vi "control gas flow.vi"(5 "gas flow, %":dbl=11.0, 6 "action":T2(ring)=enum."stop UP/DOWN", 7 "heater":dbl=11.0, 8 "gas flow":refnum<vi>, 10 "seconds":i32=1) -> (0 "gas flow out":T1={"ramp DOWN time step (sec)"=120, "DOWN step (%)"=3.0, "last check (min)"=3, "heater below"=TRUE, "heater above"=FALSE, "check every # min"=11.0, "upper"=12.0, "lower"=3.0, "heater"=0.0, "heater in range"=FALSE, "(total # of ramp DOWN steps)"=30, "ramp step (%)"=0.1, "DOWN time (min)"=60.0, "UP time (min)"=60.0, "(total # of ramp UP steps)"=30, "UP step (%)"=3.0, "ramp UP time step (sec)"=120, "set gas"=FALSE, "to"=90.0, "ramp UP"=FALSE, "ramp DOWN"=FALSE, "ramp UP steps so far"=2, "ramp UP in progress"=FALSE, "ramp DOWN steps so far "=0, "ramp DOWN in progress"=FALSE, "idle"=FALSE, "Gas flow, %"=90.0, "Control Gas"=FALSE, "state"=enum."ramp down"} {"Gas flow, %" format="%.2f"; "heater" format="%.2f"})   [LabVIEW 2010]
uses:
  gas flow control.ctl
  itc 503 box - control.ctl
panel:
  in  "gas flow control":T1={"ramp DOWN time step (sec)"=120, "DOWN step (%)"=3.0, "last check (min)"=3, "heater below"=TRUE, "heater above"=FALSE, "check every # min"=11.0, "upper"=12.0, "lower"=3.0, "heater"=0.0, "heater in range"=FALSE, "(total # of ramp DOWN steps)"=30, "ramp step (%)"=0.1, "DOWN time (min)"=60.0, "UP time (min)"=60.0, "(total # of ramp UP steps)"=30, "UP step (%)"=3.0, "ramp UP time step (sec)"=120, "set gas"=FALSE, "to"=90.0, "ramp UP"=FALSE, "ramp DOWN"=FALSE, "ramp UP steps so far"=2, "ramp UP in progress"=FALSE, "ramp DOWN steps so far "=0, "ramp DOWN in progress"=FALSE, "idle"=FALSE, "Gas flow, %"=90.0, "Control Gas"=FALSE, "state"=enum."ramp down"} {"Gas flow, %" format="%.2f"; "heater" format="%.2f"}
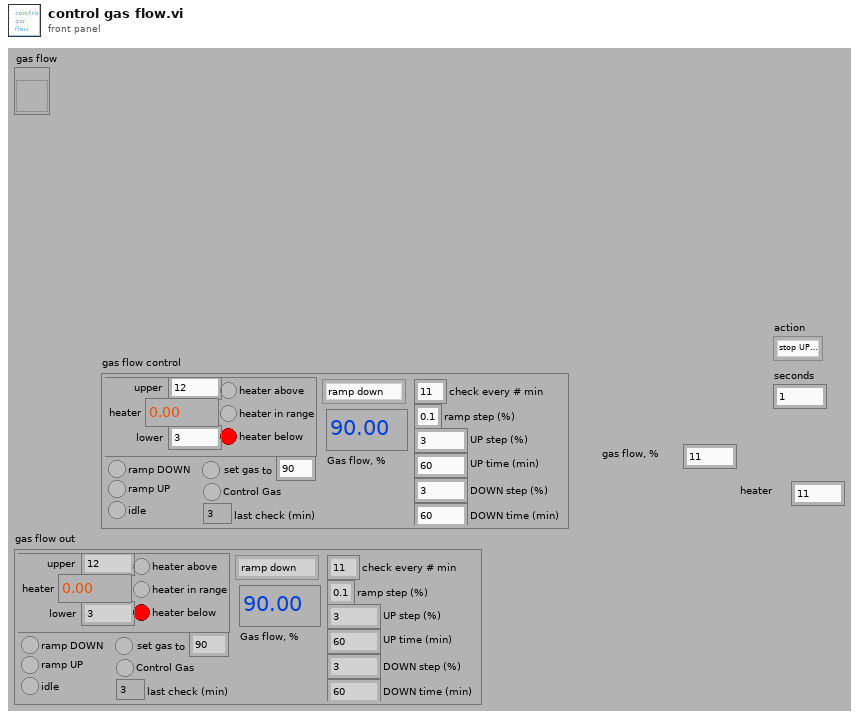
[diagram p1: front panel]
types:
  T1 = typedef "gas flow control.ctl" = cluster{"ramp DOWN time step (sec)":i32, "DOWN step (%)":dbl, "last check (min)":i32, "heater below":bool, "heater above":bool, "check every # min":dbl, "upper":dbl, "lower":dbl, "heater":dbl, "heater in range":bool, "(total # of ramp DOWN steps)":i32, "ramp step (%)":dbl, "DOWN time (min)":dbl, "UP time (min)":dbl, "(total # of ramp UP steps)":i32, "UP step (%)":dbl, "ramp UP time step (sec)":i32, "set gas":bool, "to":dbl, "ramp UP":bool, "ramp DOWN":bool, "ramp UP steps so far":i32, "ramp UP in progress":bool, "ramp DOWN steps so far ":i32, "ramp DOWN in progress":bool, "idle":bool, "Gas flow, %":dbl, "Control Gas":bool, "state":enum16{"normal", "ramp up", "ramp down"}}
  T2 = enum16{"check", "force UP", "stop UP/DOWN", "force DOWN", "init", "set gas to", "turn off", "turn on", "update parameters"}
  T3 = typedef "itc 503 box - control.ctl" = enum16{"heater manual and zero", "heater auto", "upload D", "upload I", "upload P", "shut off", "init", "read sweep table", "disable", "enable", "read state", "set gas to", "stop sweep", "start sweep", "test", "set temperature to", "write sweep table"}
  T4 = cluster{"ramp DOWN time step (sec)":i32, "DOWN step (%)":dbl, "last check (min)":i32, "heater below":bool, "heater above":bool, "check every # min":dbl, "upper":dbl, "lower":dbl, "heater":dbl, "heater in range":bool, "(total # of ramp DOWN steps)":i32, "ramp step (%)":dbl, "DOWN time (min)":dbl, "UP time (min)":dbl, "(total # of ramp UP steps)":i32, "UP step (%)":dbl, "ramp UP time step (sec)":i32, "set gas":bool, "to":dbl, "ramp UP":bool, "ramp DOWN":bool, "ramp UP steps so far":i32, "ramp UP in progress":bool, "ramp DOWN steps so far ":i32, "ramp DOWN in progress":bool, "idle":bool, "Gas flow, %":dbl, "Control Gas":bool, "state":enum16{"normal", "ramp up", "ramp down"}}
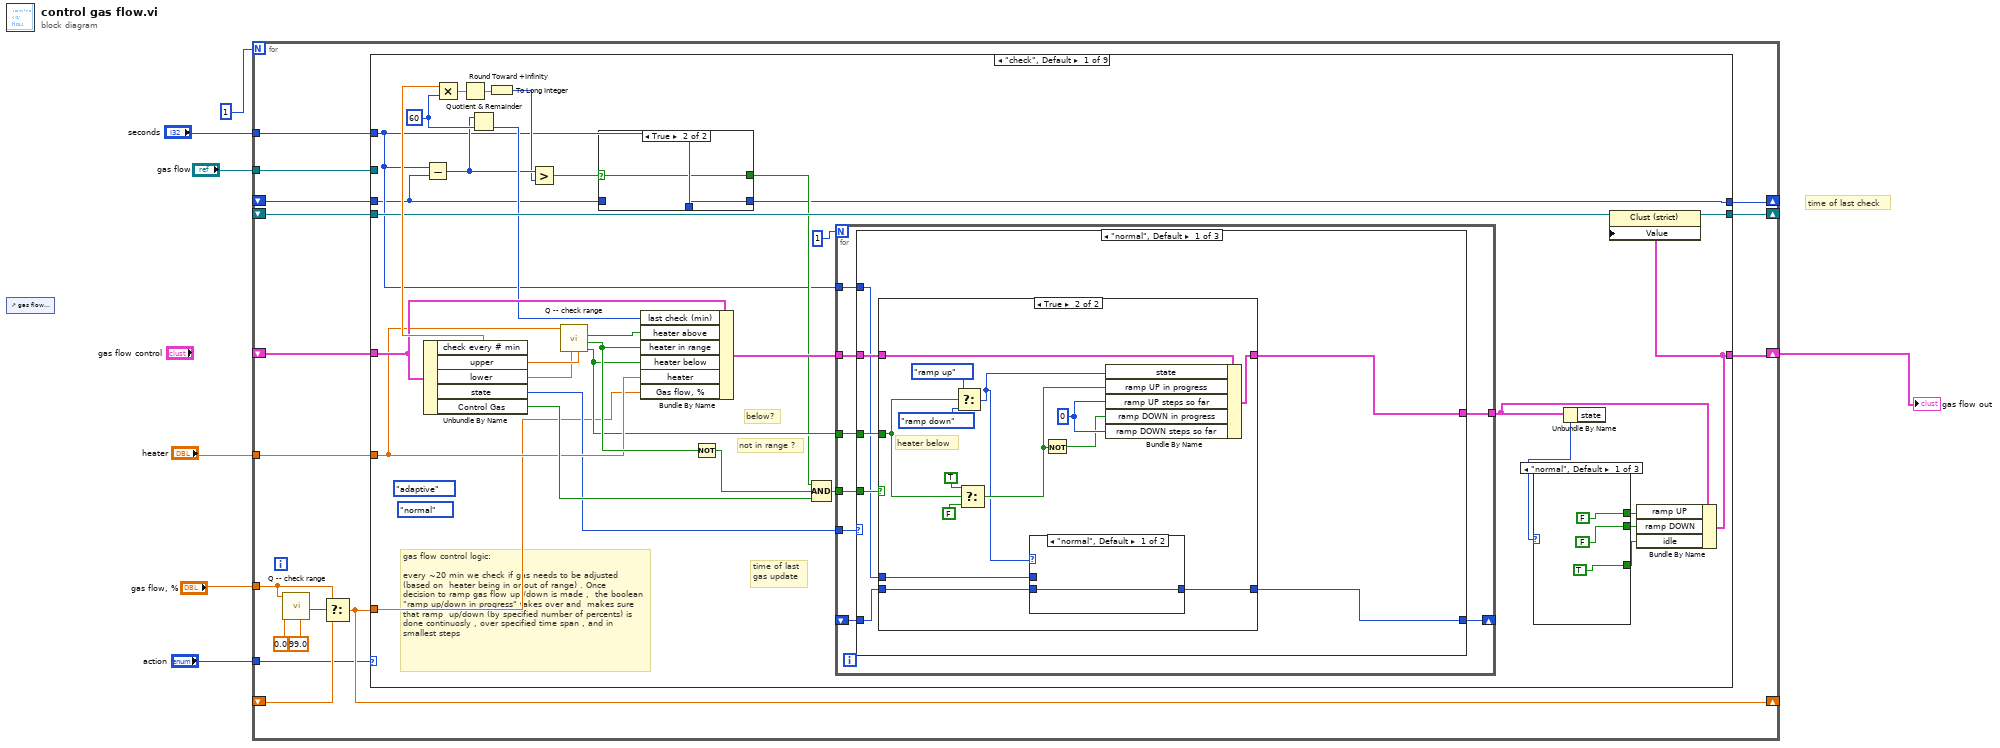
[diagram p0: block diagram]
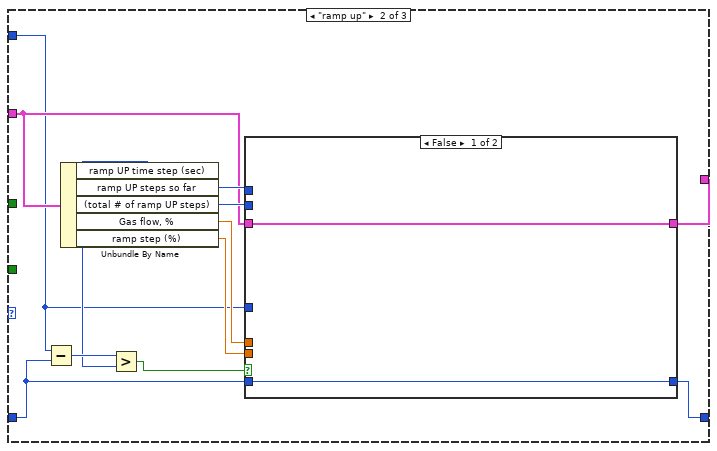
[diagram p4: hidden frame]
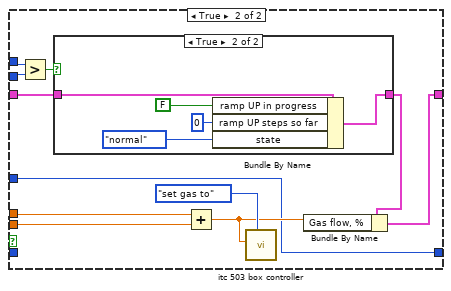
[diagram p5: hidden frame]
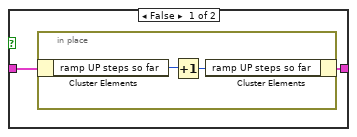
[diagram p6: hidden frame]
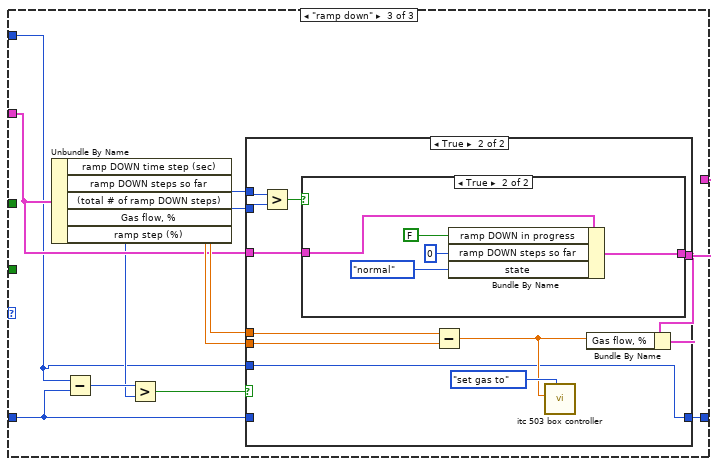
[diagram p7: hidden frame]
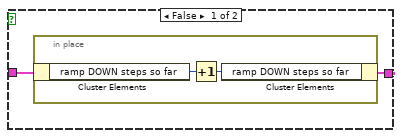
[diagram p9: hidden frame]
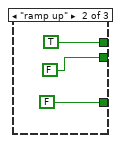
[diagram p11: hidden frame]
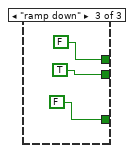
[diagram p12: hidden frame]
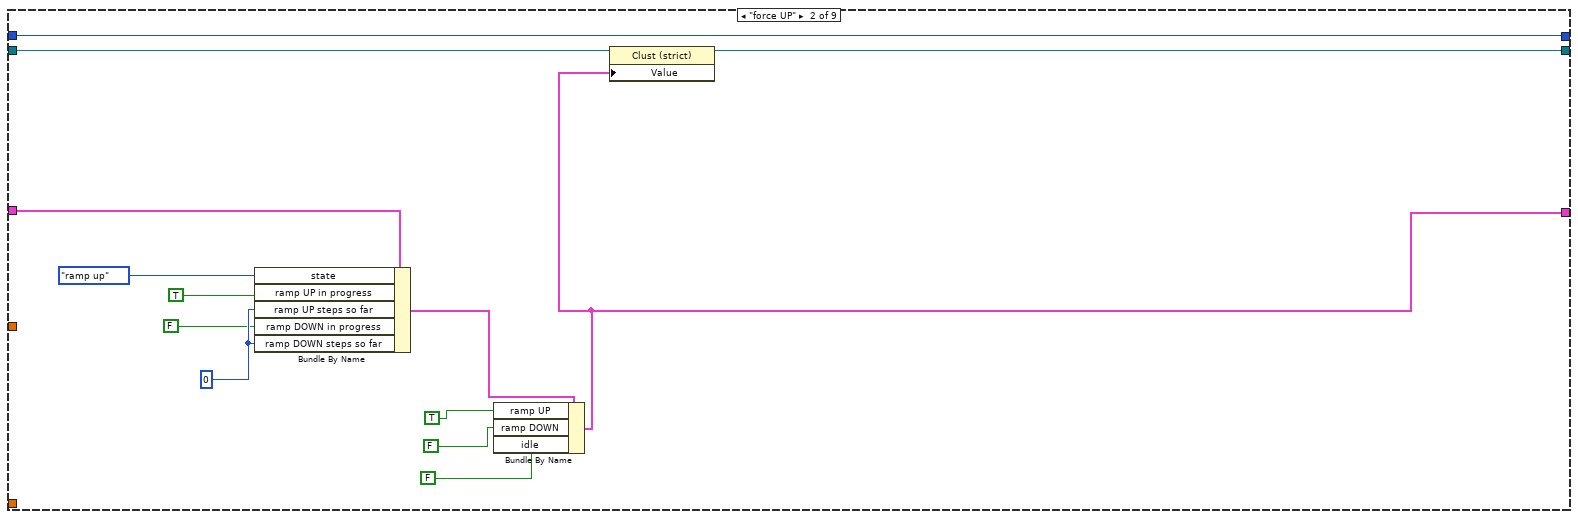
[diagram p13: hidden frame]
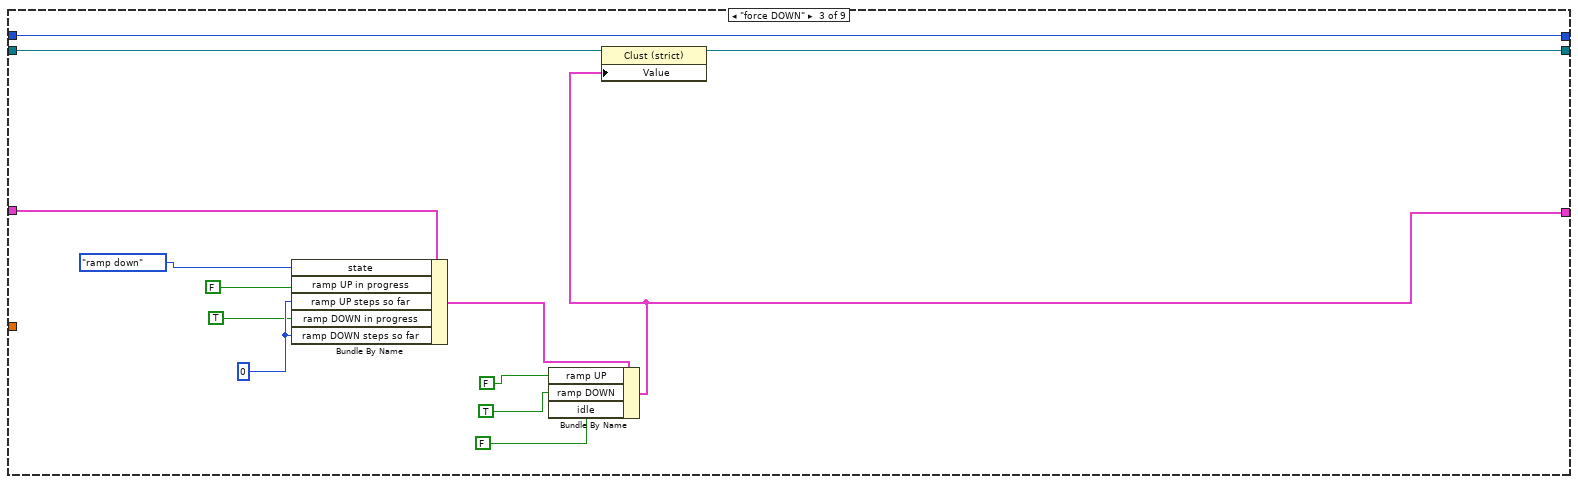
[diagram p14: hidden frame]
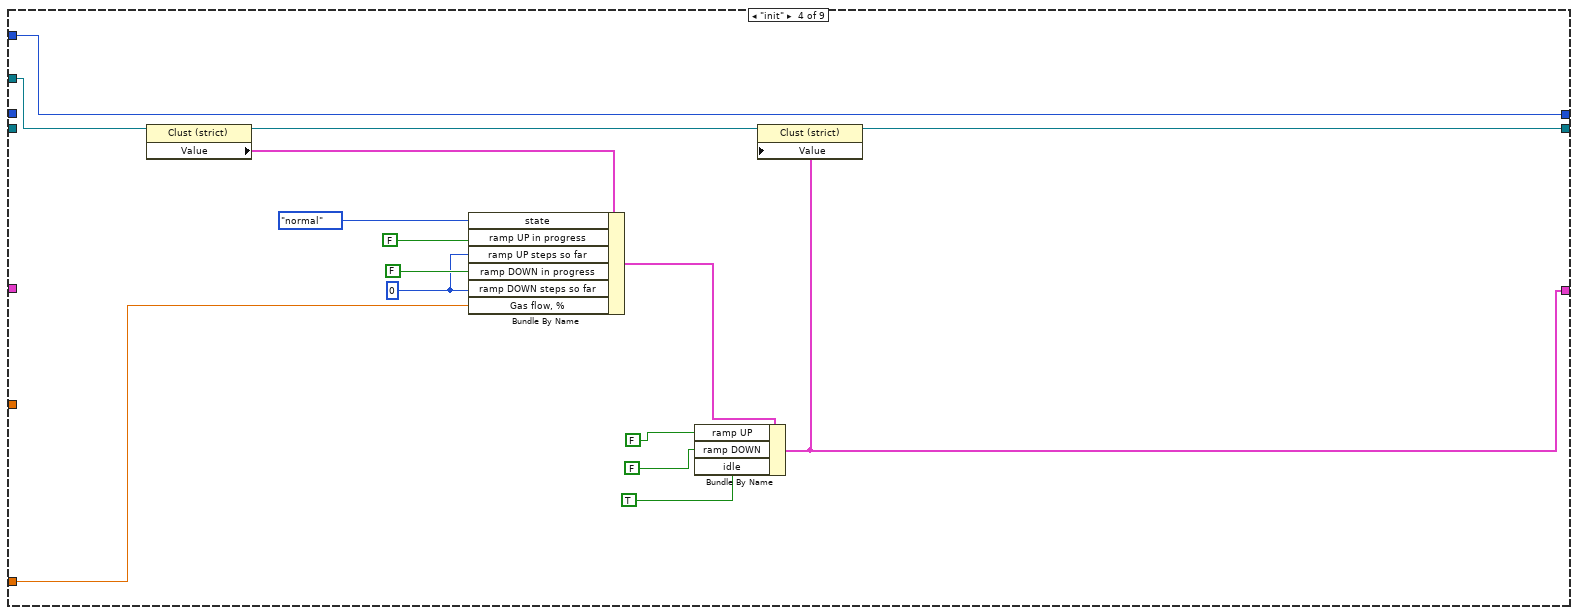
[diagram p15: hidden frame]
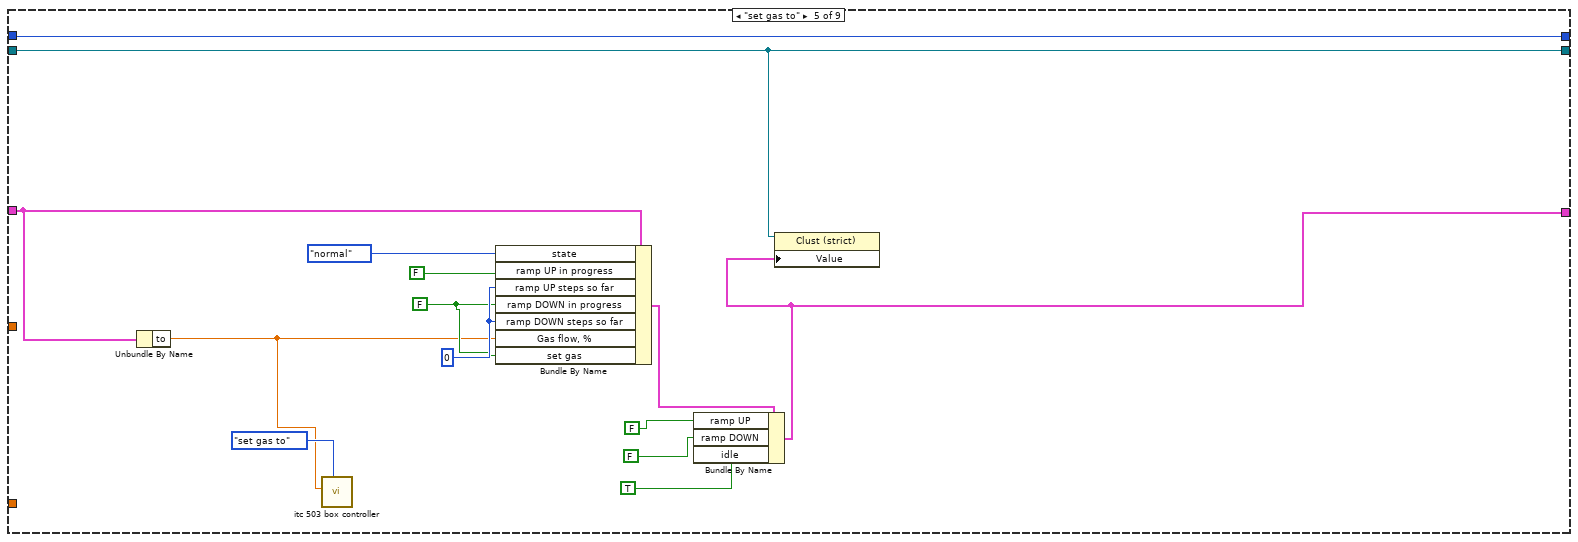
[diagram p16: hidden frame]
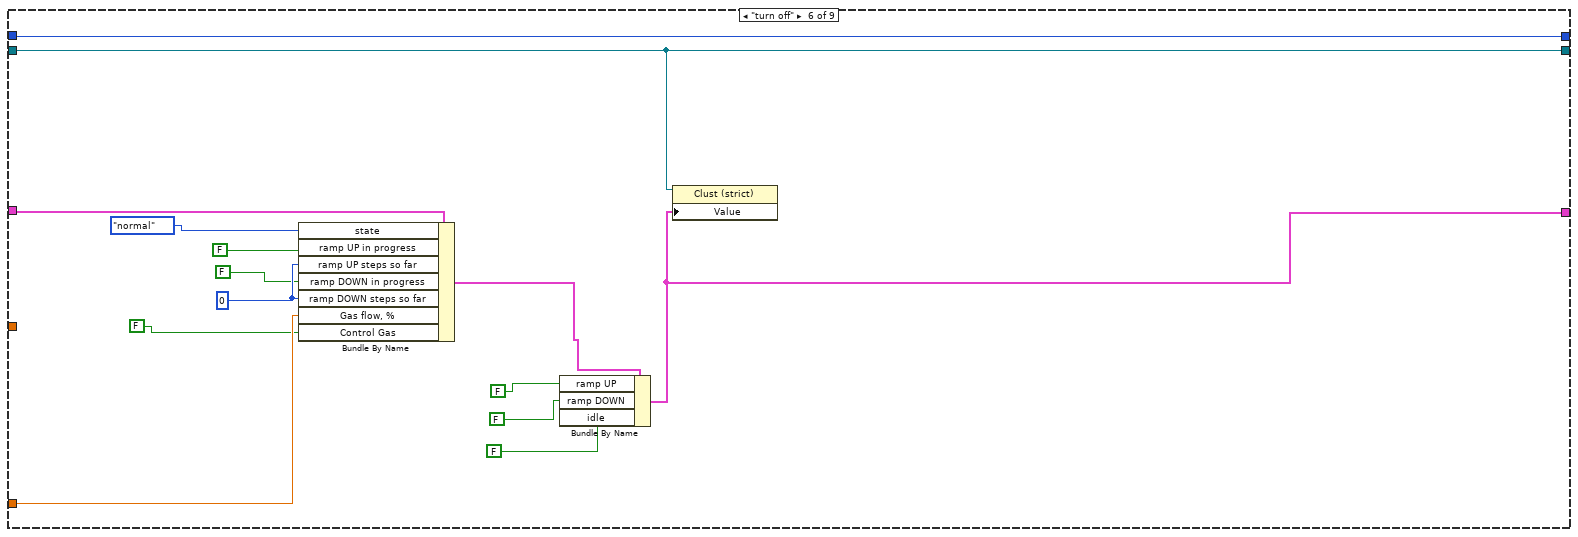
[diagram p17: hidden frame]
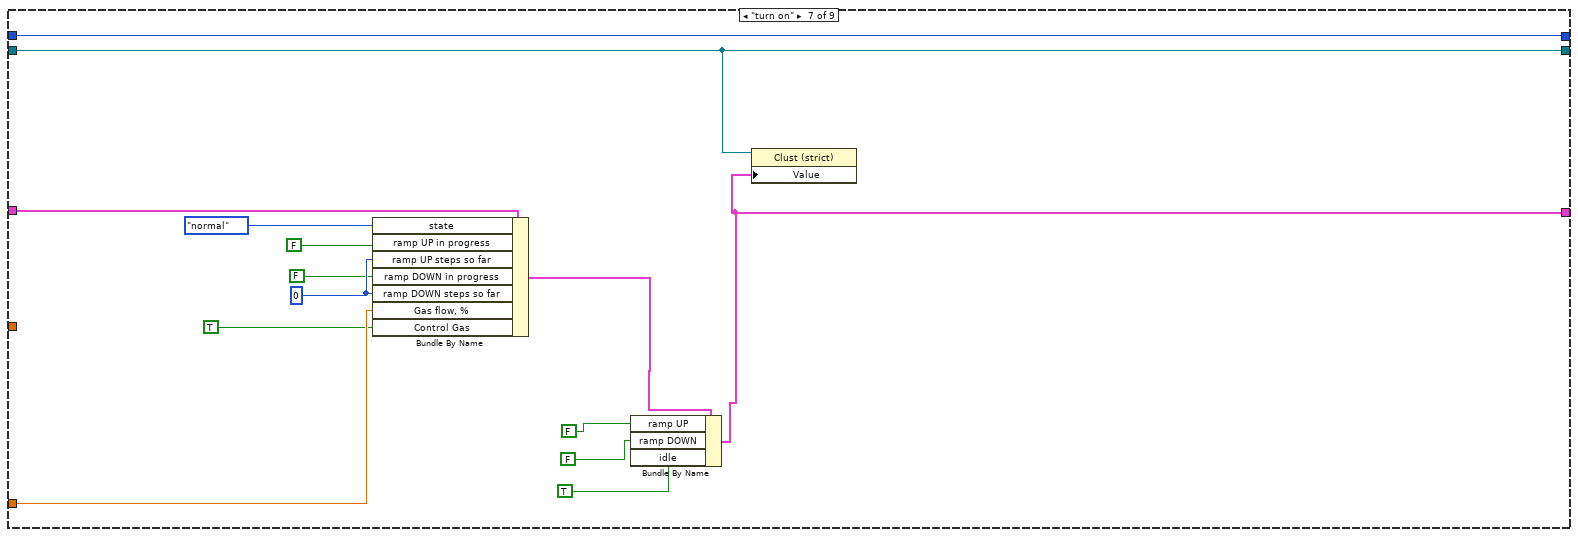
[diagram p18: hidden frame]
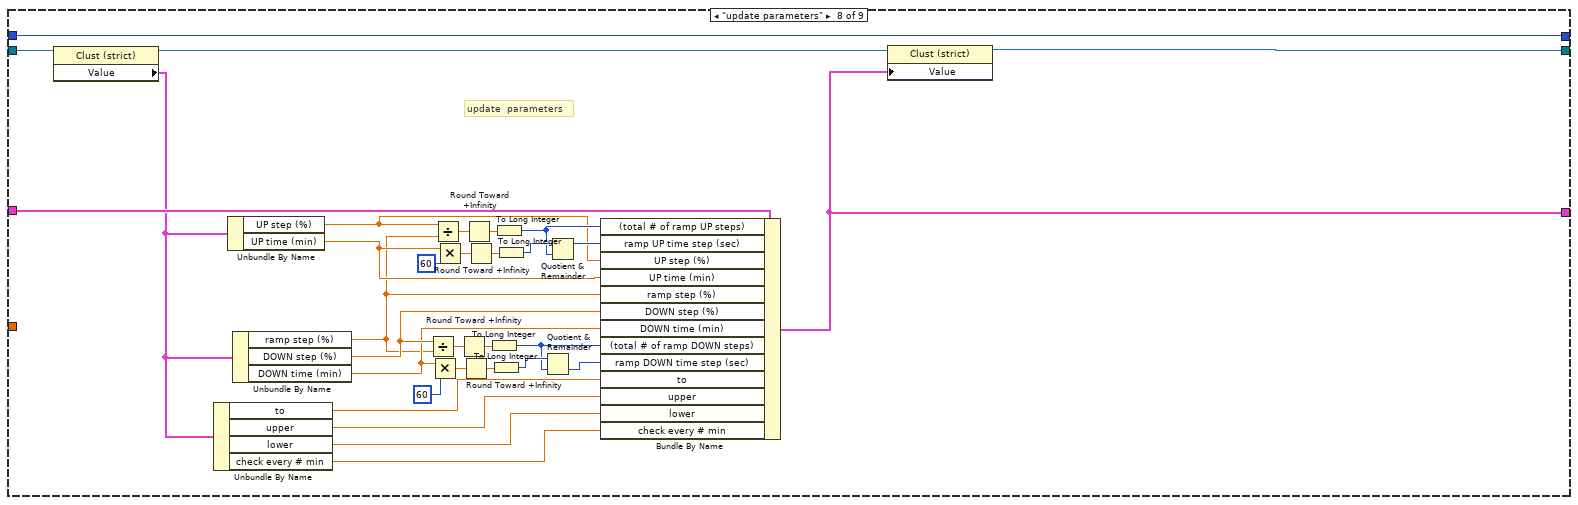
[diagram p19: hidden frame]
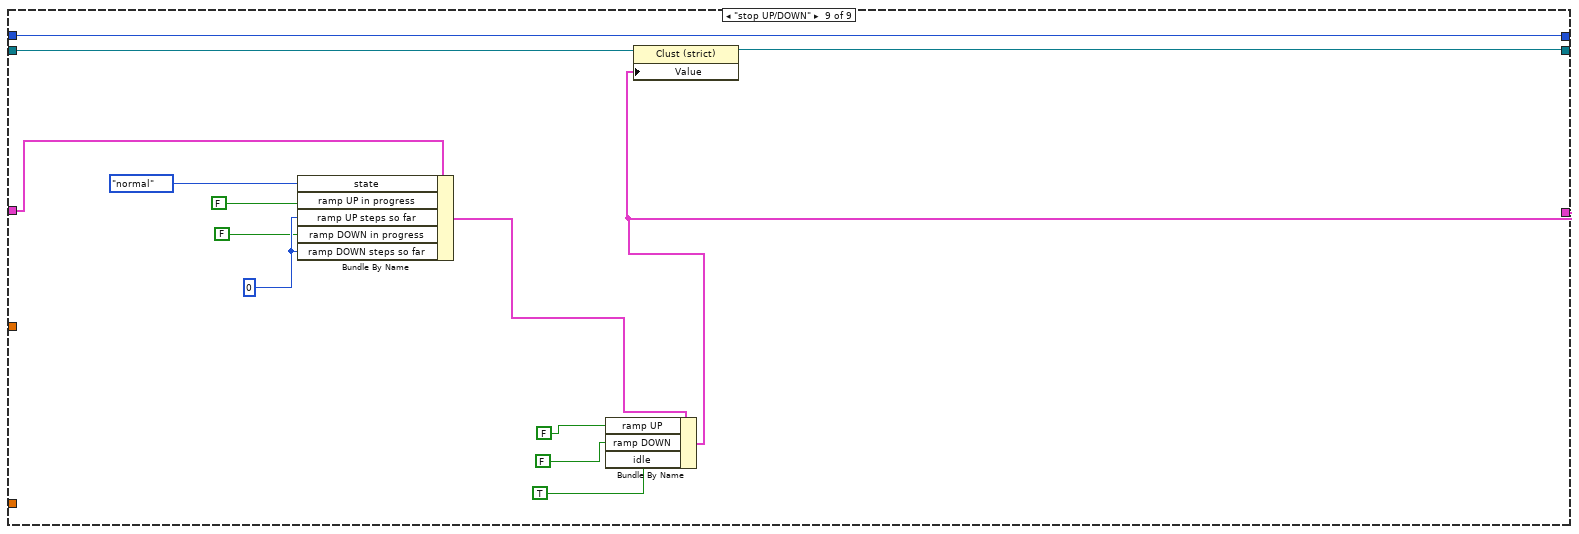
[diagram p20: hidden frame]
diagram:
  # "time of last check"
  n1 = control-ref of="gas flow control"() -> ()  [unwired: 1 out]
  n2 = for {
    N: 1 -> [_]
    shift-right: [w23] -> w2
    shift-left: _ -> [w15]
    shift-right: [w21] -> _
    shift-left: _ -> [w22]
    tunnel: "action" -> [w20]
    tunnel: "gas flow, %" -> [w16]
    tunnel: "heater" -> [w14]
    tunnel: "seconds" -> [w13]
    tunnel: "gas flow" -> [w12]
    shift-right: [w11] -> _
    shift-left: _ -> [w10]
    shift-right: [w9] -> _
    shift-left: _ -> [w8]
    n3 = call "Q -- check range.vi"("upper"=99.0 ("y"), "lower"=0.0 ("y"), "number"=w16) -> ("in range?"=w17:bool)  [unwired: 4 in, 4 out]
    n4 = Select(t=w16, s=w17, f=w22) -> (s? t:f=w21:dbl)
    n5 = case shown="\"check\", Default" w20 {
      tunnel: [w34 w177 w187 w200 w216 w228 w242 w265 w289] -> w23
      tunnel: w21 -> [w42 _ _ w209 _ w237 w251 _ _]
      tunnel: w15 -> [w47 w180 w193 _ w223 w235 w250 w271 w296]
      tunnel: w14 -> [w46 _ _ _ _ _ _ _ _]
      tunnel: w13 -> [w26 _ _ w198 _ _ _ _ _]
      tunnel: w12 -> [_ _ _ w208 _ _ _ _ _]
      tunnel: [w41 w172 w185 w205 w221 w234 w249 w259 w287] -> w11
      tunnel: w10 -> [w40 w179 w192 _ w221 w234 w249 w260 w295]
      tunnel: [w27 w173 w186 w198 w213 w227 w241 w255 w288] -> w9
      tunnel: w8 -> [w25 w173 w186 _ w213 w227 w241 w255 w288]
      frame "check", Default {
        (unwired) enum16{"normal", "ramp up", "ramp down"}."normal" ("state")
        (unwired) enum16{"first time", "uniform", "adaptive"}."adaptive" ("mode")
        w33 = 60 ("y")
        # "time of last\ngas update"
        # "gas flow control logic: \n\nevery ~20 min we check if gas needs to be adjusted  (based on  heater being in or out of range) . Once  decision to ramp gas flow up /down is made ,  the boolean \"ramp up/down in progress\" takes over and  makes sure that ramp  up/down (by specified number of percents) is done continuosly , over specified time span , and in smallest steps"
        # "not in range ?"
        # "below?"
        n6 = Unbundle By Name(w47) -> ("check every # min"=w57:dbl, "upper"=w52:dbl, "lower"=w51:dbl, "state"=w43:enum16{"normal", "ramp up", "ramp down"}, "Control Gas"=w56:bool)
        n7 = Subtract(x=w26, y=w25) -> (x-y=w31:i32)
        n8 = Multiply(x=w57, y=w33) -> (x*y=w55:dbl)
        n9 = Round Toward +Infinity(x=w55) -> (ceil(x): smallest int >= x=w54:dbl)
        n10 = Quotient & Remainder(x=w31, y=w33) -> (floor(x/y)=w32:i32)  [unwired: 1 out]
        n11 = To Long Integer(number=w54) -> (32bit integer=w30:i32)
        n12 = Greater?(x=w31, y=w30) -> (0:w29:bool)
        n13 = call "Q -- check range.vi"("upper"=w52, "lower"=w51, "number"=w46) -> ("below ?"=w44:bool, "in range?"=w49:bool, "above ?"=w50:bool)  [unwired: 4 in, 2 out]
        n14 = case shown="True" w29 {
          selector: w29 -> [w160 w162]
          tunnel: [w160 w162] -> w28
          tunnel: [w159 w161] -> w27
          tunnel: w26 -> [_ w161]
          tunnel: w25 -> [w159 _]
          frame False {
          }
          frame True {
          }
        }
        n15 = Bundle By Name(cluster=w47, "last check (min)"=w32, "heater above"=w50, "heater in range"=w49, "heater below"=w44, "heater"=w46, "Gas flow, %"=w42) -> (w48:T4)
        n16 = Not(x=w49) -> (.not. x?=w53:bool)
        n17 = Compound Arithmetic op=AND(w28, w53, w56) -> (w45:bool)
        n18 = for {
          N: 1 -> [_]
          tunnel: w48 -> [w65]
          tunnel: w45 -> [w64]
          tunnel: w44 -> [w63]
          tunnel: w43 -> [w62]
          tunnel: [w61] -> w35
          tunnel: w26 -> [w60]
          shift-right: [w59] -> _
          shift-left: _ -> [w58]
          n19 = case shown="\"normal\", Default" w62 {
            tunnel: [w70 w97 w131] -> w61
            tunnel: w65 -> [w71 w100 w132]
            tunnel: w63 -> [w72 _ _]
            tunnel: w64 -> [w69 _ _]
            tunnel: w60 -> [w68 w91 w126]
            tunnel: [w67 w94 w127] -> w59
            tunnel: w58 -> [w66 w92 w125]
            frame "normal", Default {
              n20 = case shown="True" w69 {
                tunnel: w72 -> [_ w83]
                tunnel: w71 -> [w74 w86]
                tunnel: [w74 w85] -> w70
                tunnel: w68 -> [_ w76]
                tunnel: [w73 w77] -> w67
                tunnel: w66 -> [w73 w75]
                frame False {
                }
                frame True {
                  w84 = 0 ("ramp up steps so far")
                  # "heater below"
                  n21 = Select(t=enum16{"normal", "ramp up", "ramp down"}."ramp up" ("state"), s=w83, f=enum16{"normal", "ramp up", "ramp down"}."ramp down" ("state")) -> (s? t:f=w78:enum16{"normal", "ramp up", "ramp down"})
                  n22 = Select(t=TRUE, s=w83, f=FALSE) -> (s? t:f=w80:bool)
                  n23 = case shown="\"normal\", Default" w78 {
                    tunnel: [w89 w90] -> w77
                    tunnel: w76 -> [_ w90]
                    tunnel: w75 -> [w89 _]
                    frame "normal", Default {
                    }
                    frame "ramp up", "ramp down" {
                    }
                  }
                  n24 = Not(x=w80) -> (.not. x?=w79:bool)
                  n25 = Bundle By Name(cluster=w86, "state"=w78, "ramp UP in progress"=w80, "ramp UP steps so far"=w84, "ramp DOWN in progress"=w79, "ramp DOWN steps so far"=w84) -> (w85:T4)
                }
              }
            }
            frame "ramp up" {
              n26 = Subtract(x=w91, y=w92) -> (x-y=w96:i32)
              n27 = Unbundle By Name(w100) -> ("ramp UP time step (sec)"=w93:i32, "ramp UP steps so far"=w101:i32, "(total # of ramp UP steps)"=w102:i32, "Gas flow, %"=w99:dbl, "ramp step (%)"=w98:dbl)
              n28 = Greater?(x=w96, y=w93) -> (0:w95:bool)
              n29 = case shown="False" w95 {
                tunnel: w102 -> [_ w115]
                tunnel: w101 -> [_ w114]
                tunnel: w100 -> [w104 w112]
                tunnel: [w104 w108] -> w97
                tunnel: w99 -> [_ w111]
                tunnel: w98 -> [_ w110]
                tunnel: [w103 w105] -> w94
                tunnel: w91 -> [_ w105]
                tunnel: w92 -> [w103 _]
                frame False {
                }
                frame True {
                  n30 = Greater?(x=w114, y=w115) -> (0:w113:bool)
                  n31 = case shown="True" w113 {
                    tunnel: w112 -> [w117 w124]
                    tunnel: [w116 w120] -> w109
                    frame False {
                      n32 = in-place {
                        n33 = in-place-cluster #1(w117) -> ("ramp UP steps so far"=w119:i32)
                        n34 = Increment(x=w119) -> (x+1=w118:i32)
                        n35 = in-place-cluster #1("ramp UP steps so far"=w118) -> (w116:T4)
                      }
                    }
                    frame True {
                      n36 = Bundle By Name(cluster=w124, "ramp UP in progress"=FALSE, "ramp UP steps so far"=0 ("ramp up steps so far"), "state"=enum16{"normal", "ramp up", "ramp down"}."normal") -> (w120:T4)
                    }
                  }
                  n37 = Add(x=w111, y=w110) -> (x+y=w106:dbl)
                  n38 = call "itc 503 box controller.vi"("itc box action"=itc_503_box_-_control."set gas to", "input"=w106) -> ()  [unwired: 7 in, 3 out]
                  n39 = Bundle By Name(cluster=w109, "Gas flow, %"=w106) -> (w108:T4)
                }
              }
            }
            frame "ramp down" {
              n40 = Unbundle By Name(w132) -> ("ramp DOWN time step (sec)"=w128:i32, "ramp DOWN steps so far"=w135:i32, "(total # of ramp DOWN steps)"=w136:i32, "Gas flow, %"=w134:dbl, "ramp step (%)"=w133:dbl)
              n41 = Subtract(x=w126, y=w125) -> (x-y=w130:i32)
              n42 = Greater?(x=w130, y=w128) -> (0:w129:bool)
              n43 = case shown="True" w129 {
                tunnel: w136 -> [_ w149]
                tunnel: w135 -> [_ w148]
                tunnel: w132 -> [w138 w146]
                tunnel: [w138 w142] -> w131
                tunnel: w134 -> [_ w145]
                tunnel: w133 -> [_ w144]
                tunnel: [w137 w139] -> w127
                tunnel: w126 -> [_ w139]
                tunnel: w125 -> [w137 _]
                frame False {
                }
                frame True {
                  n44 = Greater?(x=w148, y=w149) -> (0:w147:bool)
                  n45 = case shown="True" w147 {
                    tunnel: w146 -> [w151 w158]
                    tunnel: [w150 w155] -> w143
                    frame False {
                      n46 = in-place {
                        n47 = in-place-cluster #2(w151) -> ("ramp DOWN steps so far"=w153:i32)
                        n48 = Increment(x=w153) -> (x+1=w152:i32)
                        n49 = in-place-cluster #2("ramp DOWN steps so far"=w152) -> (w150:T4)
                      }
                    }
                    frame True {
                      n50 = Bundle By Name(cluster=w158, "ramp DOWN in progress"=FALSE, "ramp DOWN steps so far"=0 ("ramp up steps so far"), "state"=enum16{"normal", "ramp up", "ramp down"}."normal") -> (w155:T4)
                    }
                  }
                  n51 = Subtract(x=w145, y=w144) -> (x-y=w140:dbl)
                  n52 = call "itc 503 box controller.vi"("itc box action"=itc_503_box_-_control."set gas to", "input"=w140) -> ()  [unwired: 7 in, 3 out]
                  n53 = Bundle By Name(cluster=w143, "Gas flow, %"=w140) -> (w142:T4)
                }
              }
            }
          }
        }
        n54 = Unbundle By Name(w35) -> ("state"=w39:enum16{"normal", "ramp up", "ramp down"})
        n55 = case shown="\"normal\", Default" w39 {
          tunnel: [FALSE TRUE FALSE] -> w38
          tunnel: [FALSE FALSE TRUE] -> w37
          tunnel: [TRUE FALSE FALSE] -> w36
          frame "normal", Default {
          }
          frame "ramp up" {
          }
          frame "ramp down" {
          }
        }
        n56 = Bundle By Name(cluster=w35, "ramp UP"=w38, "ramp DOWN"=w37, "idle"=w36) -> (w34:T4)
        n57 = property class="Clust (strict)"(reference=w40, "Value"=w34) -> (reference out=w41:refnum<vi>)  [unwired: 1 in, 1 out]
      }
      frame "force UP" {
        w184 = 0 ("ramp up steps so far")
        n58 = Bundle By Name(cluster=w180, "state"=enum16{"normal", "ramp up", "ramp down"}."ramp up", "ramp UP in progress"=TRUE, "ramp UP steps so far"=w184, "ramp DOWN in progress"=FALSE, "ramp DOWN steps so far"=w184) -> (w178:T4)
        n59 = Bundle By Name(cluster=w178, "ramp UP"=TRUE, "ramp DOWN"=FALSE, "idle"=FALSE) -> (w177:T4)
        n60 = property class="Clust (strict)"(reference=w179, "Value"=w177) -> (reference out=w172:refnum<vi>)  [unwired: 1 in, 1 out]
      }
      frame "force DOWN" {
        w197 = 0 ("ramp up steps so far")
        n61 = Bundle By Name(cluster=w193, "state"=enum16{"normal", "ramp up", "ramp down"}."ramp down", "ramp UP in progress"=FALSE, "ramp UP steps so far"=w197, "ramp DOWN in progress"=TRUE, "ramp DOWN steps so far"=w197) -> (w188:T4)
        n62 = Bundle By Name(cluster=w188, "ramp UP"=FALSE, "ramp DOWN"=TRUE, "idle"=FALSE) -> (w187:T4)
        n63 = property class="Clust (strict)"(reference=w192, "Value"=w187) -> (reference out=w185:refnum<vi>)  [unwired: 1 in, 1 out]
      }
      frame "init" {
        w199 = 0 ("ramp up steps so far")
        n64 = property class="Clust (strict)"(reference=w208) -> (reference out=w206:refnum<vi>, "Value"=w207:T4)  [unwired: 1 in, 1 out]
        n65 = Bundle By Name(cluster=w207, "state"=enum16{"normal", "ramp up", "ramp down"}."normal", "ramp UP in progress"=FALSE, "ramp UP steps so far"=w199, "ramp DOWN in progress"=FALSE, "ramp DOWN steps so far"=w199, "Gas flow, %"=w209) -> (w201:T4)
        n66 = Bundle By Name(cluster=w201, "ramp UP"=FALSE, "ramp DOWN"=FALSE, "idle"=TRUE) -> (w200:T4)
        n67 = property class="Clust (strict)"(reference=w206, "Value"=w200) -> (reference out=w205:refnum<vi>)  [unwired: 1 in, 1 out]
      }
      frame "set gas to" {
        w222 = FALSE
        w226 = 0 ("ramp up steps so far")
        n68 = Unbundle By Name(w223) -> ("to"=w214:dbl)
        n69 = call "itc 503 box controller.vi"("itc box action"=itc_503_box_-_control."set gas to", "input"=w214) -> ()  [unwired: 7 in, 3 out]
        n70 = Bundle By Name(cluster=w223, "state"=enum16{"normal", "ramp up", "ramp down"}."normal", "ramp UP in progress"=FALSE, "ramp UP steps so far"=w226, "ramp DOWN in progress"=w222, "ramp DOWN steps so far"=w226, "Gas flow, %"=w214, "set gas"=w222) -> (w217:T4)
        n71 = Bundle By Name(cluster=w217, "ramp UP"=FALSE, "ramp DOWN"=FALSE, "idle"=TRUE) -> (w216:T4)
        n72 = property class="Clust (strict)"(reference=w221, "Value"=w216) -> ()  [unwired: 1 in, 2 out]
      }
      frame "turn off" {
        w240 = 0 ("ramp up steps so far")
        n73 = Bundle By Name(cluster=w235, "state"=enum16{"normal", "ramp up", "ramp down"}."normal", "ramp UP in progress"=FALSE, "ramp UP steps so far"=w240, "ramp DOWN in progress"=FALSE, "ramp DOWN steps so far"=w240, "Gas flow, %"=w237, "Control Gas"=FALSE) -> (w229:T4)
        n74 = Bundle By Name(cluster=w229, "ramp UP"=FALSE, "ramp DOWN"=FALSE, "idle"=FALSE) -> (w228:T4)
        n75 = property class="Clust (strict)"(reference=w234, "Value"=w228) -> ()  [unwired: 1 in, 2 out]
      }
      frame "turn on" {
        w254 = 0 ("ramp up steps so far")
        n76 = Bundle By Name(cluster=w250, "state"=enum16{"normal", "ramp up", "ramp down"}."normal", "ramp UP in progress"=FALSE, "ramp UP steps so far"=w254, "ramp DOWN in progress"=FALSE, "ramp DOWN steps so far"=w254, "Gas flow, %"=w251, "Control Gas"=TRUE) -> (w243:T4)
        n77 = Bundle By Name(cluster=w243, "ramp UP"=FALSE, "ramp DOWN"=FALSE, "idle"=TRUE) -> (w242:T4)
        n78 = property class="Clust (strict)"(reference=w249, "Value"=w242) -> ()  [unwired: 1 in, 2 out]
      }
      frame "update parameters" {
        # "update  parameters"
        n79 = property class="Clust (strict)"(reference=w260) -> (reference out=w272:refnum<vi>, "Value"=w264:T4)  [unwired: 1 in, 1 out]
        n80 = Unbundle By Name(w264) -> ("to"=w263:dbl, "upper"=w262:dbl, "lower"=w261:dbl, "check every # min"=w258:dbl)
        n81 = Unbundle By Name(w264) -> ("UP step (%)"=w256:dbl, "UP time (min)"=w270:dbl)
        n82 = Unbundle By Name(w264) -> ("ramp step (%)"=w257:dbl, "DOWN step (%)"=w269:dbl, "DOWN time (min)"=w268:dbl)
        n83 = Divide(x=w269, y=w257) -> (x/y=w278:dbl)
        n84 = Multiply(x=w268, y=60) -> (x*y=w276:dbl)
        n85 = Divide(x=w256, y=w257) -> (x/y=w286:dbl)
        n86 = Multiply(x=w270, y=60) -> (x*y=w284:dbl)
        n87 = Round Toward +Infinity(x=w278) -> (ceil(x): smallest int >= x=w277:dbl)
        n88 = Round Toward +Infinity(x=w276) -> (ceil(x): smallest int >= x=w275:dbl)
        n89 = Round Toward +Infinity(x=w286) -> (ceil(x): smallest int >= x=w285:dbl)
        n90 = Round Toward +Infinity(x=w284) -> (ceil(x): smallest int >= x=w283:dbl)
        n91 = To Long Integer(number=w277) -> (32bit integer=w266:i32)
        n92 = To Long Integer(number=w275) -> (32bit integer=w273:i32)
        n93 = To Long Integer(number=w285) -> (32bit integer=w280:i32)
        n94 = To Long Integer(number=w283) -> (32bit integer=w281:i32)
        n95 = Quotient & Remainder(x=w273, y=w266) -> (floor(x/y)=w267:i32)  [unwired: 1 out]
        n96 = Quotient & Remainder(x=w281, y=w280) -> (floor(x/y)=w279:i32)  [unwired: 1 out]
        n97 = Bundle By Name(cluster=w271, "(total # of ramp UP steps)"=w280, "ramp UP time step (sec)"=w279, "UP step (%)"=w256, "UP time (min)"=w270, "ramp step (%)"=w257, "DOWN step (%)"=w269, "DOWN time (min)"=w268, "(total # of ramp DOWN steps)"=w266, "ramp DOWN time step (sec)"=w267, "to"=w263, "upper"=w262, "lower"=w261, "check every # min"=w258) -> (w265:T4)
        n98 = property class="Clust (strict)"(reference=w272, "Value"=w265) -> (reference out=w259:refnum<vi>)  [unwired: 1 in, 1 out]
      }
      frame "stop UP/DOWN" {
        w299 = 0 ("ramp up steps so far")
        n99 = Bundle By Name(cluster=w296, "state"=enum16{"normal", "ramp up", "ramp down"}."normal", "ramp UP in progress"=FALSE, "ramp UP steps so far"=w299, "ramp DOWN in progress"=FALSE, "ramp DOWN steps so far"=w299) -> (w290:T4)
        n100 = Bundle By Name(cluster=w290, "ramp UP"=FALSE, "ramp DOWN"=FALSE, "idle"=TRUE) -> (w289:T4)
        n101 = property class="Clust (strict)"(reference=w295, "Value"=w289) -> (reference out=w287:refnum<vi>)  [unwired: 1 in, 1 out]
      }
    }
  }
  "gas flow out" <- w2
